vi "TopoG_Supply.vi"() -> ()   [LabVIEW 2019]
uses:
  <userlib>/_TI-LA/Instr Drivers/Power Supply/E3631/Driver/EasyIO/Typedefs/E3631 Output States.ctl
  <userlib>/_TI-LA/Instr Drivers/Power Supply/E3631/Driver/EasyIO/Typedefs/E3631 Output State.ctl
  <userlib>/_TI-LA/Instr Drivers/Power Supply/E3631/Driver/EasyIO/Typedefs/E3631 Channel Selection.ctl
  <userlib>/_TI-LA/Instr Drivers/Power Supply/E3631/Driver/EasyIO/Typedefs/E3631 Outputs Settings.ctl
  <userlib>/_TI-LA/Instr Drivers/Power Supply/E3631/Driver/EasyIO/Typedefs/E3631 Output Configuration.ctl
  <userlib>/_TI-LA/Instr Drivers/Power Supply/E3631/Driver/EasyIO/Typedefs/E3631 Action.ctl
  <userlib>/_TI-LA/Instr Drivers/Power Supply/E3631/Driver/EasyIO/Typedefs/E3631 OP State.ctl
  <userlib>/_TI-LA/Instr Drivers/Power Supply/E3631/Driver/E3631.lvlib
panel:
  in  "Enum":enum16{"Configure", "Output_State"}(ring)=enum."Output_State"
  in  "ID Query (T: Check) 2":bool=TRUE
  in  "Tab Control 2":T1(tab)
  in  "E363x outputs settings 2":T2={"Channel 1 (+6V)"={"action"=enum."Configure channel", "voltage (V)"=1.22, "current limit (A)"=0.02, "Enable?"=TRUE}, "Channel 2 (+25V)"={"action"=enum."Configure channel", "voltage (V)"=3.3, "current limit (A)"=0.07, "Enable?"=TRUE}, "Channel 3 (-25V)"={"action"=enum."Keep current settings", "voltage (V)"=0.0, "current limit (A)"=nan, "Enable?"=TRUE}} {"Channel 3 (-25V)"."current limit (A)" min=0.0 max=1.0 step=0.25 format="%.3p"; "Channel 3 (-25V)"."voltage (V)" min=-25.0 max=25.0 step=0.25 format="%.3p"; "Channel 2 (+25V)"."current limit (A)" min=0.0 max=1.0 step=0.25 format="%.3p"; "Channel 2 (+25V)"."voltage (V)" min=-25.0 max=25.0 step=0.25 format="%.3p"; "Channel 1 (+6V)"."current limit (A)" min=0.0 max=1.0 step=0.25 format="%.3p"; "Channel 1 (+6V)"."voltage (V)" min=-25.0 max=25.0 step=0.25 format="%.3p"}
  in  "Channel Selection for Readback 2":T5={"Channel 1"=TRUE, "Channel 2"=TRUE, "Channel 3"=TRUE}
  in  "Read Output? 2":bool=TRUE
  out "E363x outputs states 2":T6 {"Channel3"."Actual Current (A)" format="%.3p"; "Channel3"."Actual Voltage (V)" format="%.3p"; "Channel2"."Actual Current (A)" format="%.3p"; "Channel2"."Actual Voltage (V)" format="%.3p"; "Channel1"."Actual Current (A)" format="%.3p"; "Channel1"."Actual Voltage (V)" format="%.3p"}
  in  "MCU_Supply":refnum<visa-resource-name>="GPIB0::5::INSTR"
  in  "Reset 1":bool
  in  "ID Query (T: Check)":bool=TRUE
  in  "Tab Control":T1(tab)
  in  "E363x outputs settings":T2={"Channel 1 (+6V)"={"action"=enum."Configure channel", "voltage (V)"=5.0, "current limit (A)"=0.08, "Enable?"=TRUE}, "Channel 2 (+25V)"={"action"=enum."Configure channel", "voltage (V)"=5.0, "current limit (A)"=0.07, "Enable?"=TRUE}, "Channel 3 (-25V)"={"action"=enum."Configure channel", "voltage (V)"=-5.0, "current limit (A)"=0.07, "Enable?"=TRUE}} {"Channel 3 (-25V)"."current limit (A)" min=0.0 max=1.0 step=0.25 format="%.3p"; "Channel 3 (-25V)"."voltage (V)" min=-25.0 max=25.0 step=0.25 format="%.3p"; "Channel 2 (+25V)"."current limit (A)" min=0.0 max=1.0 step=0.25 format="%.3p"; "Channel 2 (+25V)"."voltage (V)" min=-25.0 max=25.0 step=0.25 format="%.3p"; "Channel 1 (+6V)"."current limit (A)" min=0.0 max=1.0 step=0.25 format="%.3p"; "Channel 1 (+6V)"."voltage (V)" min=-25.0 max=25.0 step=0.25 format="%.3p"}
  in  "Channel Selection for Readback":T5={"Channel 1"=TRUE, "Channel 2"=TRUE, "Channel 3"=TRUE}
  in  "Read Output?":bool=TRUE
  out "E363x outputs states":T6 {"Channel3"."Actual Current (A)" format="%.3p"; "Channel3"."Actual Voltage (V)" format="%.3p"; "Channel2"."Actual Current (A)" format="%.3p"; "Channel2"."Actual Voltage (V)" format="%.3p"; "Channel1"."Actual Current (A)" format="%.3p"; "Channel1"."Actual Voltage (V)" format="%.3p"}
  in  "output state":T8=enum."ON"
  in  "Supply_505V":refnum<visa-resource-name>="GPIB0::2::INSTR"
  in  "Reset":bool
  # "Output Settings"
  # "Output Settings"
  # "Output Settings"
  # "Output Settings"
  # "Output Settings"
  # "Output Settings"
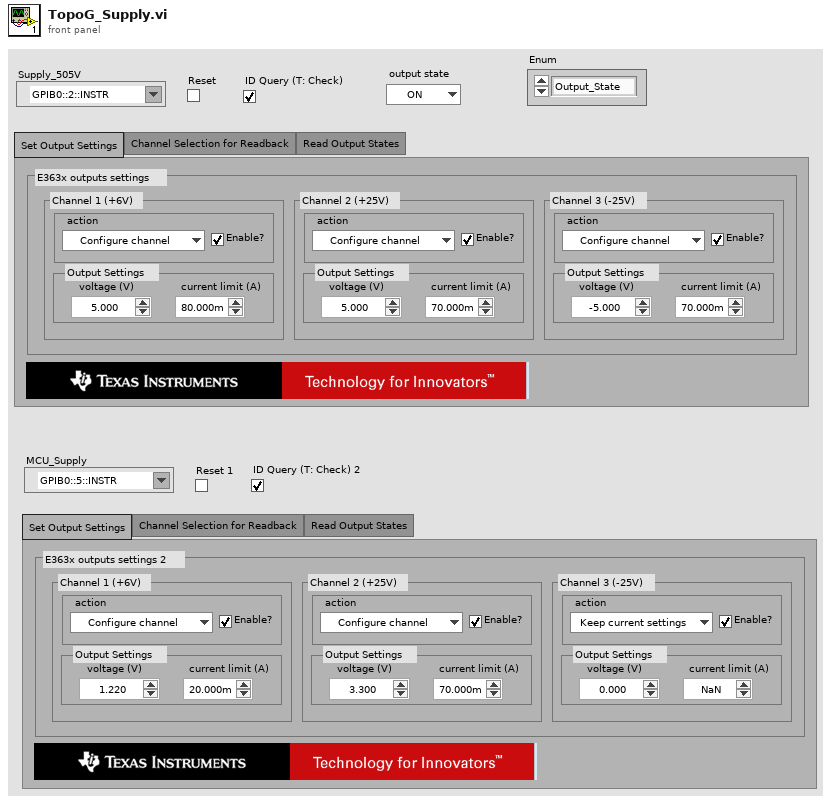
[diagram p1: front panel]
types:
  T1 = enum32{"Set Output Settings", "Channel Selection for Readback", "Read Output States"}
  T2 = typedef "E3631.lvlib/E3631 Outputs Settings.ctl" = cluster{"Channel 1 (+6V)":T3, "Channel 2 (+25V)":T3, "Channel 3 (-25V)":T3}
  T3 = typedef "E3631.lvlib/E3631 Output Configuration.ctl" = cluster{"action":T4, "voltage (V)":dbl, "current limit (A)":dbl, "Enable?":bool}
  T4 = typedef "E3631.lvlib/E3631 Action.ctl" = enum16{"Configure channel", "Keep current settings"}
  T5 = typedef "E3631.lvlib/E3631 Channel Selection.ctl" = cluster{"Channel 1":bool, "Channel 2":bool, "Channel 3":bool}
  T6 = typedef "E3631.lvlib/E3631 Output States.ctl" = cluster{"Channel1":T7, "Channel2":T7, "Channel3":T7, "Output State":bool}
  T7 = typedef "E3631.lvlib/E3631 Output State.ctl" = cluster{"Actual Voltage (V)":dbl, "Actual Current (A)":dbl}
  T8 = typedef "E3631.lvlib/E3631 OP State.ctl" = enum16{"OFF", "ON"}
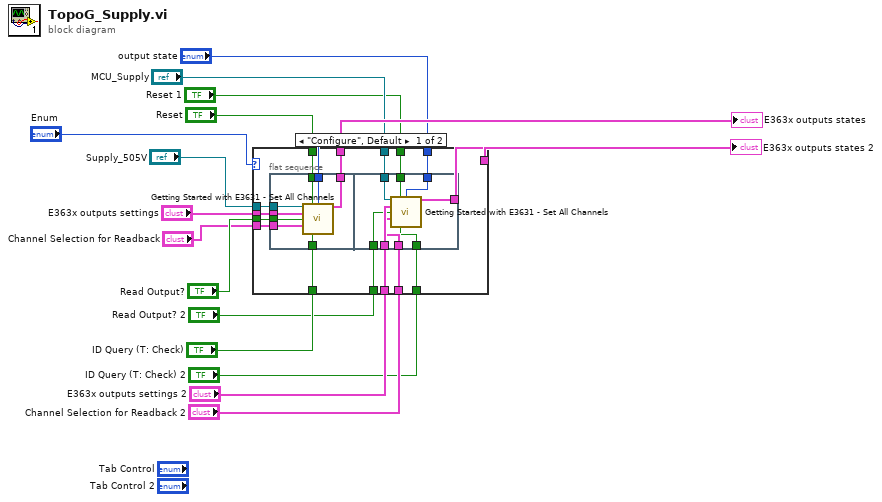
[diagram p0: block diagram]
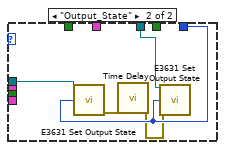
[diagram p2: hidden frame]
diagram:
  n1 = case shown="\"Configure\", Default" "Enum" {
    tunnel: "E363x outputs settings" -> [w31 _]
    tunnel: "Supply_505V" -> [w30 w52]
    tunnel: "Read Output?" -> [w29 _]
    tunnel: "ID Query (T: Check)" -> [w28 _]
    tunnel: "Reset" -> [w27 _]
    tunnel: "Channel Selection for Readback" -> [w26 _]
    tunnel: [w25 _] -> w10
    tunnel: "MCU_Supply" -> [w24 w51]
    tunnel: "Reset 1" -> [w23 _]
    tunnel: "output state" -> [w22 w50]
    tunnel: "E363x outputs settings 2" -> [w21 _]
    tunnel: "Read Output? 2" -> [w20 _]
    tunnel: "Channel Selection for Readback 2" -> [w19 _]
    tunnel: "ID Query (T: Check) 2" -> [w18 _]
    tunnel: [w17 _] -> w2
    frame "Configure", Default {
      n2 = flat-sequence {
        tunnel: w31 -> [w39]
        tunnel: w30 -> [w38]
        tunnel: w29 -> [w37]
        tunnel: w28 -> [w36]
        tunnel: w27 -> [w35]
        tunnel: w22 -> [w34]
        tunnel: w26 -> [w33]
        tunnel: [w32] -> w25
        tunnel: w24 -> [w47]
        tunnel: w23 -> [w46]
        tunnel: w22 -> [w45]
        tunnel: w21 -> [w44]
        tunnel: w20 -> [w43]
        tunnel: w19 -> [w42]
        tunnel: w18 -> [w41]
        tunnel: [w40] -> w17
        frame #0 {
          n3 = call <userlib>:"Getting Started with E3631 - Set All Channels.vi"("Instrument handle In"=w38, "Reset"=w35, "output state"=w34, "E363x outputs settings"=w39, "Read Output?"=w37, "Channel Selection for Readback"=w33, "ID Query (T: Check)"=w36) -> ("E363x outputs states"=w32:T6)  [unwired: 8 in]
        }
        frame #1 {
          n4 = call <userlib>:"Getting Started with E3631 - Set All Channels.vi"("Instrument handle In"=w47, "Reset"=w46, "output state"=w45, "E363x outputs settings"=w44, "Read Output?"=w43, "Channel Selection for Readback"=w42, "ID Query (T: Check)"=w41) -> ("E363x outputs states"=w40:T6)  [unwired: 8 in]
        }
      }
    }
    frame "Output_State" {
      n5 = call <userlib>:"E3631 Set Output State.vi"("VISA session"=w52, "Output state"=w50) -> ("error out"=w48:errorcluster)  [unwired: 3 in, 10 out]
      n6 = call "Time Delay"("error in (no error)"=w48) -> ("error out"=w49:errorcluster)  [unwired: 10 in]
      n7 = call <userlib>:"E3631 Set Output State.vi"("VISA session"=w51, "Output state"=w50, "error in"=w49) -> ()  [unwired: 2 in, 11 out]
    }
  }
  "E363x outputs states" <- w10
  "E363x outputs states 2" <- w2
